vi "MQTT_Simple_Connect_and_Publish.vi"() -> ()   [LabVIEW 2015, in "MQTT_Functions.lvlib"]
doc: "A simple client example that connects to a broker server and publishes messages to a topic.\n\n© 2015 - daq.io, LLC - Peter Adelhardt MQTT LabVIEW Client 0.9.0.3\nPeter Adelhardt - daq.io\nCopyright (c) 2016, daq.io"
uses:
  <vilib>/daq.io/MQTT LabVIEW Client/MQTT_Functions.lvlib
  <vilib>/daq.io/MQTT LabVIEW Client/Controls/QoS.ctl
  <vilib>/daq.io/MQTT LabVIEW Client/Controls/Retain_Flag.ctl
  <vilib>/daq.io/MQTT LabVIEW Client/Controls/DUP_Flag.ctl
  <vilib>/daq.io/MQTT LabVIEW Client/Controls/Connection_Return_Codes.ctl
  <vilib>/daq.io/MQTT LabVIEW Client/Controls/Connect_Flags.ctl
panel:
  out "Message published":string
  in  "Stop Publishing":bool
  out "Message ID (acknowledged)":u16=10
  out "Acknowledged":bool
  in  "Message ID":u16=20
  in  "MQTT Broker":cluster{"address (IP)":string, "port":u16}={"address (IP)"="212.72.74.21", "port"=1883}
  in  "Message to be published":string="LabVIEW says it's "
  out "Connection Status":T1=enum."Connection refused: not authorized"
  out "error out":errorcluster
  in  "Client ID":string="androidTest"
  in  "error in (no error)":errorcluster
  in  "Topic":string="androidTest"
  in  "Publish Meta":cluster{"QoS":T2, "Retain":T3, "DUP":T4}
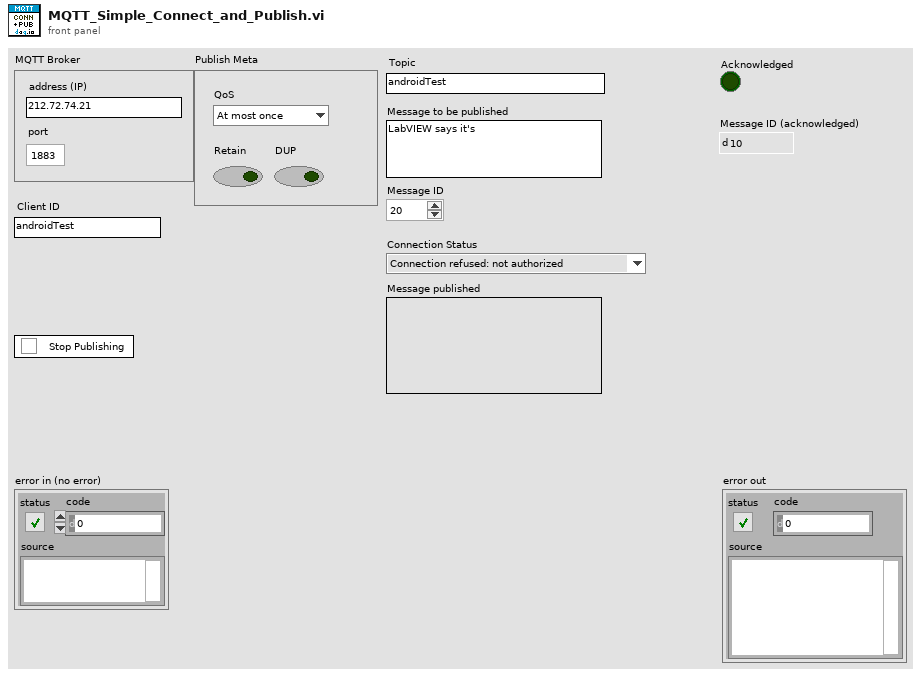
[diagram p1: front panel]
types:
  T1 = typedef "MQTT_Functions.lvlib/Connection_Return_Codes.ctl" = enum16{"Connection accepted", "Connection refused: unacceptable protocol version", "Connection refused: identifier rejected", "Connection refused: Server unavailable", "Connection refused: bad user name or password", "Connection refused: not authorized"}
  T2 = typedef "MQTT_Functions.lvlib/QoS.ctl" = enum8{"At most once", "At least once", "Exactly once", "Reserved"}
  T3 = typedef "MQTT_Functions.lvlib/Retain_Flag.ctl" = bool
  T4 = typedef "MQTT_Functions.lvlib/DUP_Flag.ctl" = bool
  T5 = typedef "MQTT_Functions.lvlib/Connect_Flags.ctl" = cluster{"user name":bool, "password":bool, "will retain":bool, "will flag":bool, "clean session":bool, "reserved":bool, "will QoS":T2}
  T6 = cluster{"QoS":T2, "DUP":T4, "Retain":T3, "Keep Alive (sec)":u16}
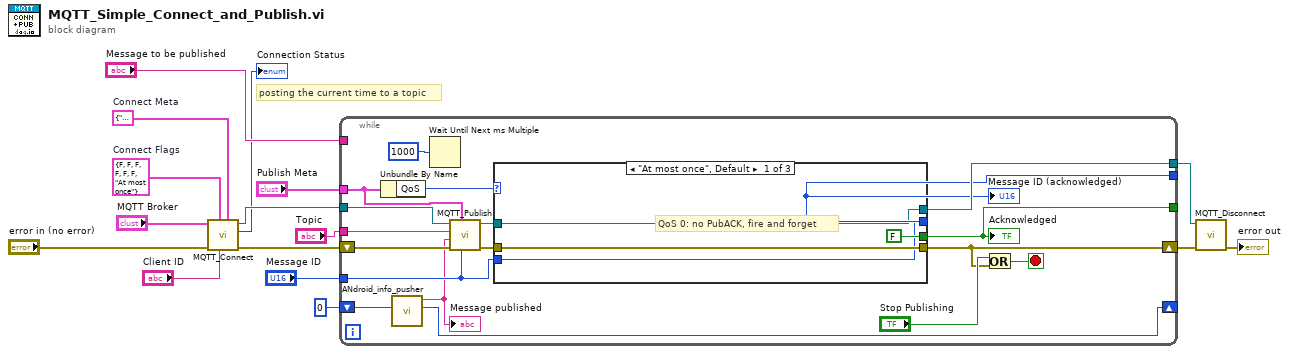
[diagram p0: block diagram]
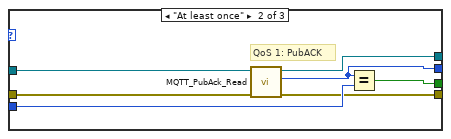
[diagram p2: hidden frame]
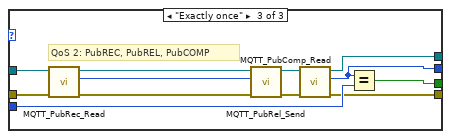
[diagram p3: hidden frame]
diagram:
  w14 = T5 {"user name"=FALSE, "password"=FALSE, "will retain"=FALSE, "will flag"=FALSE, "clean session"=FALSE, "reserved"=FALSE, "will QoS"=enum."At most once"}  # Connect Flags
  w11 = T6 {"QoS"=enum."At most once", "DUP"=FALSE, "Retain"=FALSE, "Keep Alive (sec)"=60}  # Connect Meta
  # "posting the current time to a topic"
  n1 = call <vilib>:"MQTT_Connect.vi"("Connect Meta"=w11, "Client ID"="Client ID", "Connect Flags"=w14, "error in (no error)"="error in (no error)", "MQTT Broker"="MQTT Broker") -> ("error out"=w2:errorcluster, "Connection Status"=→"Connection Status":T1, "connection ID out"=w4:refnum<k5>)  [unwired: 4 in]
  n2 = while {
    tunnel: "Topic" -> [w34]
    tunnel: "Message to be published" -> [_]
    tunnel: w4 -> [w33]
    tunnel: "Publish Meta" -> [w31]
    tunnel: [w27] -> w7
    tunnel: "Message ID" -> [w26]
    tunnel: [w21] -> _
    tunnel: [w20] -> _
    shift-right: [w23] -> w8
    shift-left: w2 -> [w32]
    shift-right: [w18] -> _
    shift-left: 0 -> [w17]
    stop <- w24 stop-if-true
    n3 = Unbundle By Name(w31) -> ("QoS"=w30:T2)
    n4 = call "ANdroid_info_pusher.vi"("IndexerIn"=w17) -> ("indexout"=w18:i32, "spreadsheet string"=w19:string)  [unwired: 9 in]
    "Message published" <- w19
    n5 = Wait Until Next ms Multiple(millisecond multiple=u32 1000) -> ()  [unwired: 1 out]
    n6 = call <vilib>:"MQTT_Publish.vi"("Message ID"=w26, "Publish Meta"=w31, "error in (no error)"=w32, "Message to be published"=w19, "Topic"=w34, "connection ID"=w33) -> ("error out"=w29:errorcluster, "connection ID out"=w28:refnum<k5>)  [unwired: 4 in]
    n7 = case shown="\"At most once\", Default" w30 {
      tunnel: w29 -> [w37 w44 w56]
      tunnel: w28 -> [w38 w45 w57]
      tunnel: [w37 w42 w49] -> w23
      tunnel: [w38 w41 w50] -> w27
      tunnel: w26 -> [w35 w43 w55]
      tunnel: [FALSE w40 w51] -> w21
      tunnel: [w35 w39 w48] -> w20
      frame "At most once", Default {
        # "QoS 0: no PubACK, fire and forget"
      }
      frame "At least once" {
        # "QoS 1: PubACK"
        n8 = call <vilib>:"MQTT_PubAck_Read.vi"("error in (no error)"=w44, "connection ID"=w45) -> ("error out"=w42:errorcluster, "Message ID"=w39:u16, "connection ID out"=w41:refnum<k5>)  [unwired: 7 in]
        n9 = Equal?(x=w39, y=w43) -> (x = y?=w40:bool)
      }
      frame "Exactly once" {
        # "QoS 2: PubREC, PubREL, PubCOMP"
        n10 = call <vilib>:"MQTT_PubRec_Read.vi"("error in (no error)"=w56, "connection ID"=w57) -> ("error out"=w54:errorcluster, "Message ID"=w52:u16, "connection ID out"=w53:refnum<k5>)  [unwired: 7 in]
        n11 = call <vilib>:"MQTT_PubRel_Send.vi"("error in (no error)"=w54, "Message ID"=w52, "connection ID"=w53) -> ("error out"=w46:errorcluster, "connection ID out"=w47:refnum<k5>)  [unwired: 6 in, 1 out]
        n12 = call <vilib>:"MQTT_PubComp_Read.vi"("error in (no error)"=w46, "connection ID"=w47) -> ("error out"=w49:errorcluster, "Message ID"=w48:u16, "connection ID out"=w50:refnum<k5>)  [unwired: 7 in]
        n13 = Equal?(x=w48, y=w55) -> (x = y?=w51:bool)
      }
    }
    "Message ID (acknowledged)" <- w20
    "Acknowledged" <- w21
    n14 = Or(x="Stop Publishing", y=w23) -> (x .or. y?=w24:bool)
  }
  n15 = call <vilib>:"MQTT_Disconnect.vi"("error in (no error)"=w8, "connection ID"=w7) -> ("error out"=→"error out":errorcluster)  [unwired: 9 in]
